vi "Get Node Attributes.vi"(8 "error in (no error)":errorcluster, 10 "names":string[](array[string]), 11 "node in":refnum<k20>) -> (0 "error out":errorcluster, 2 "values":string[](array[string]), 3 "node out":refnum<k20>)   [LabVIEW 2017, in "Error File Management.lvlib"]
uses:
  Error File Management.lvlib
  <vilib>/xml/Close Reference(Node).vi
  <vilib>/xml/Close Reference(NNMap).vi
  <resource>/objmgr/DOMUserDefRef.rc
  <vilib>/xml/NI_XML.lvlib
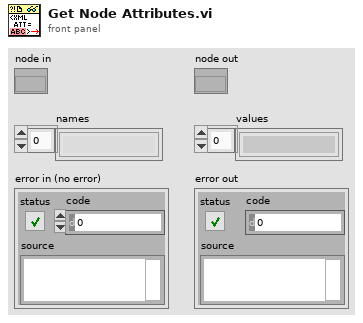
[diagram p1: front panel]
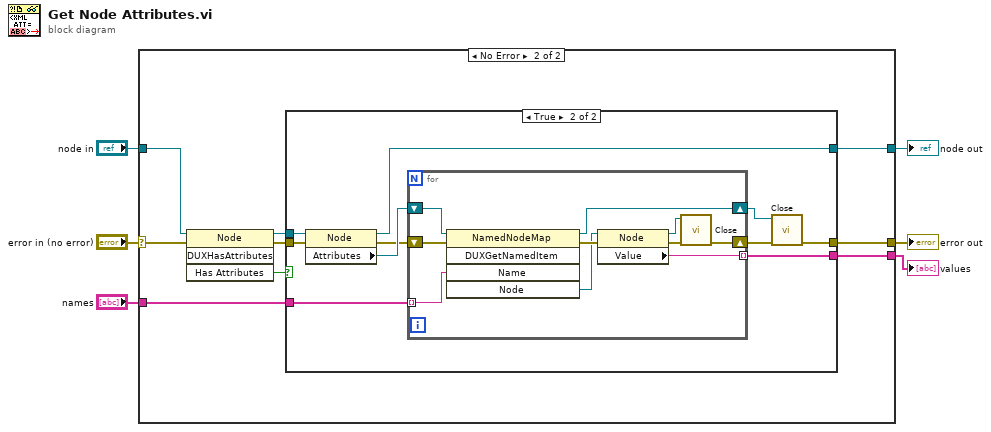
[diagram p0: block diagram]
diagram:
  n1 = case shown="No Error" "error in (no error)" {
    selector: "error in (no error)" -> [w8 w11]
    tunnel: "names" -> [_ w14]
    tunnel: [_ w13] -> w5
    tunnel: [w8 w12] -> w3
    tunnel: "node in" -> [w7 w10]
    tunnel: [w7 w9] -> w1
    frame Error {
    }
    frame No Error {
      n2 = invoke class="Node" method="DUXHasAttributes"(reference=w10, error in=w11) -> (reference out=w17:refnum<k20>, error out=w16:errorcluster, "Has Attributes"=w15:bool)  [unwired: 2 in, 1 out]
      n3 = case shown="True" w15 {
        tunnel: w17 -> [w18 w28]
        tunnel: w16 -> [w19 w27]
        tunnel: w14 -> [_ w26]
        tunnel: [_ w25] -> w13
        tunnel: [w19 w21] -> w12
        tunnel: [w18 w20] -> w9
        frame False {
        }
        frame True {
          n4 = property class="Node"(reference=w28, error in=w27) -> (reference out=w20:refnum<k20>, error out=w22:errorcluster, "Attributes"=w29:refnum<k20>)
          n5 = for {
            tunnel: w26 -> [w34] mode=indexing
            tunnel: [w33] -> w25 mode=indexing
            shift-right: [w32] -> w24
            shift-left: w22 -> [w31]
            shift-right: [w30] -> w23
            shift-left: w29 -> [w35]
            n6 = invoke class="NamedNodeMap" method="DUXGetNamedItem"(reference=w35, error in=w31, "Name"=w34) -> (reference out=w30:refnum<k20>, error out=w37:errorcluster, "Node"=w36:refnum<k20>)  [unwired: 2 in, 2 out]
            n7 = property class="Node"(reference=w36, error in=w37) -> (reference out=w39:refnum<k20>, error out=w38:errorcluster, "Value"=w33:string)
            n8 = call-poly <vilib>:"Close.vi"("error in (no error)"=w38, "node"=w39) -> ("error out"=w32:errorcluster)  [unwired: 7 out]
          }
          n9 = call-poly <vilib>:"Close.vi"("error in (no error)"=w24, "named node map"=w23) -> ("error out"=w21:errorcluster)  [unwired: 7 out]
        }
      }
    }
  }
  "values" <- w5
  "error out" <- w3
  "node out" <- w1
